vi "NF LI56xx dvr DATA POINt.vi"(8 "error in":errorcluster caption="error in (no error)" {"code" format="%.0x"}, 9 "Read(F)":bool, 10 "set buffer":enum16{"BUF1", "BUF2", "BUF3"}(ring), 11 "VISA resource name":refnum<visa-resource-name>) -> (0 "error out":errorcluster {"code" format="%.0x"}, 2 "query buffer size":string, 3 "VISA resource name copy":refnum<visa-resource-name>)   [LabVIEW 2019]
doc: "Sets/queries measurement data buffer size. \nWhen size is set, the specified measurement data buffer is cleared. \nSize is specified in sample points."
panel:
  in  "set buffer size":u32=16 min=16 max=65536 step=1
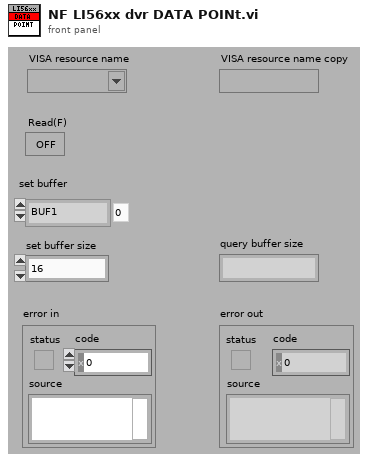
[diagram p1: front panel]
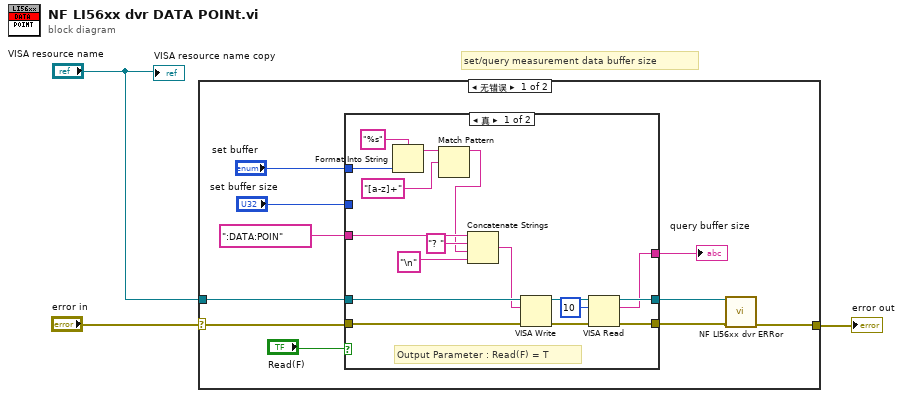
[diagram p0: block diagram]
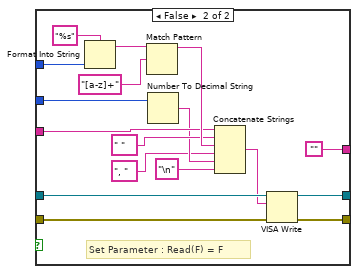
[diagram p2: hidden frame]
diagram:
  # "set/query measurement data buffer size"
  n1 = case shown="无错误" "error in" {
    selector: "error in" -> [w12 w48]
    tunnel: [w6 w48] -> w3
    tunnel: "VISA resource name" -> [w11 _]
    frame No Error {
      n2 = case shown="真" "Read(F)" {
        tunnel: w11 -> [w30 w47]
        tunnel: [w27 w44] -> w8
        tunnel: [w26 w45] -> w7
        tunnel: w12 -> [w25 w46]
        tunnel: [w21 ""] -> w10
        tunnel: "set buffer" -> [w16 w40]
        tunnel: ":DATA:POIN" ("•¶Žš—ñ") -> [w20 w36]
        tunnel: "set buffer size" -> [_ w33]
        frame True {
          # "Output Parameter : Read(F) = T"
          n3 = Format Into String(format string="%s", w16) -> (resulting string=w18:string)  [unwired: 2 in, 1 out]
          n4 = Match Pattern(string=w18, regular expression="[a-z]+") -> (before substring=w15:string)  [unwired: 1 in, 3 out]
          n5 = Concatenate Strings(w20, "? " ("Œ`Ž®•¶Žš—ñ"), w15, "\n" ("Œ`Ž®•¶Žš—ñ")) -> (w22:string)
          n6 = VISA Write(VISA resource name=w30, write buffer=w22, error in (no error)=w25) -> (VISA resource name out=w28:refnum<visa-resource-name>, error out=w29:errorcluster)  [unwired: 1 out]
          n7 = VISA Read(VISA resource name=w28, byte count=u32 10 ("バイトカウント（0）"), error in (no error)=w29) -> (VISA resource name out=w27:refnum<visa-resource-name>, read buffer=w21:string, error out=w26:errorcluster)  [unwired: 1 out]
        }
        frame False {
          # "Set Parameter : Read(F) = F"
          n8 = Format Into String(format string="%s", w40) -> (resulting string=w39:string)  [unwired: 2 in, 1 out]
          n9 = Match Pattern(string=w39, regular expression="[a-z]+") -> (before substring=w38:string)  [unwired: 1 in, 3 out]
          n10 = Number To Decimal String(number=w33) -> (decimal integer string=w32:string)  [unwired: 1 in]
          n11 = Concatenate Strings(w36, " ", w38, ", ", w32, "\n" ("Œ`Ž®•¶Žš—ñ")) -> (w42:string)
          n12 = VISA Write(VISA resource name=w47, write buffer=w42, error in (no error)=w46) -> (VISA resource name out=w44:refnum<visa-resource-name>, error out=w45:errorcluster)  [unwired: 1 out]
        }
      }
      "query buffer size" <- w10
      n13 = call "NF LI56xx dvr ERRor.vi"("VISA resource name"=w8, "error in (no error)"=w7) -> ("error out"=w6:errorcluster)  [unwired: 10 in, 3 out]
    }
    frame Error {
    }
  }
  "error out" <- w3
  "VISA resource name copy" <- "VISA resource name"
